vi "Read Controller Enqueuer.vi"(11 "Cooler":refnum<class "Cooler.lvclass">) -> (2 "Controller Enqueuer":refnum<class "Message Enqueuer.lvclass">)   [LabVIEW 2018, in "Cooler.lvlib" / "Cooler.lvclass"]
doc: "Reads the enqueuer used to send messages to the controller actor. This VI may return a Not A Refnum enqueuer because the cooler may not be controlled by any controller at the moment."
uses:
  Cooler.lvclass
  <vilib>/ActorFramework/Message Enqueuer/Message Enqueuer.lvclass
  Cooler.lvclass/Cooler.ctl
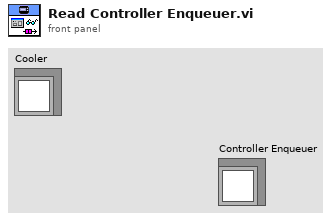
[diagram p1: front panel]
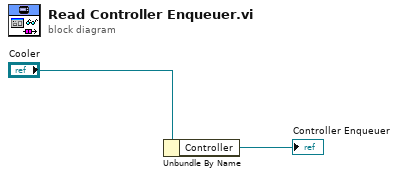
[diagram p0: block diagram]
diagram:
  n1 = Unbundle By Name("Cooler") -> ("Controller"=→"Controller Enqueuer":refnum<class "Message Enqueuer.lvclass">)
